vi "纳清电导率_所有参数读取.vi"(8 "error in (no error)":errorcluster caption="错误输入（无错误）", 11 "MB session in":refnum<class "MB_Master.lvclass">) -> (0 "error out":errorcluster caption="错误输出", 2 "输出值":T1 {"波特率" items=["4800", "9600", "19200", "38400", "57600", "115200"]}, 3 "MB session out":refnum<class "MB_Master.lvclass">)   [LabVIEW 2016, in "斯坦道多参数.lvlib"]
uses:
  <vilib>/Plasmionique/MB Master/MB_Master/MB_Master.lvclass
  <vilib>/Plasmionique/MB Master/MB Master.lvlib
  <vilib>/ptbypt/NI_PtbyPt.lvlib
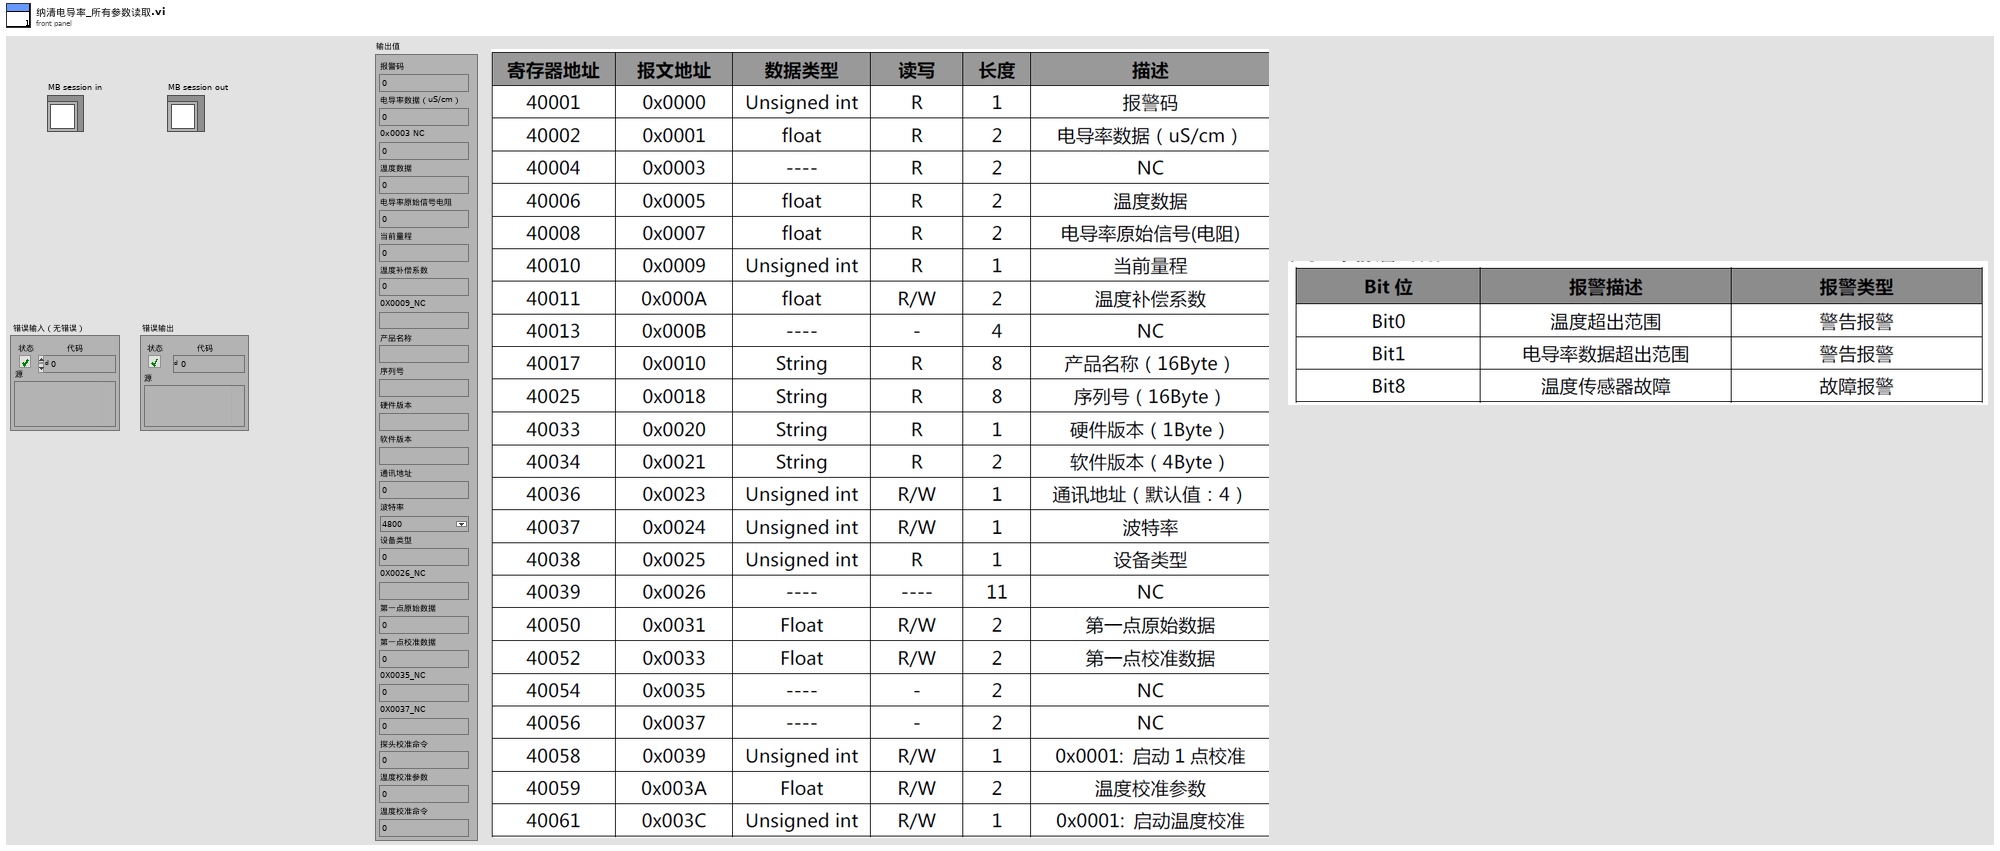
[diagram p1: front panel]
types:
  T1 = cluster{"报警码":u16, "电导率数据（uS/cm）":sgl, "0x0003 NC":sgl, "温度数据":sgl, "电导率原始信号电阻":sgl, "当前量程":u16, "温度补偿系数":sgl, "0X0009_NC":string, "产品名称":string, "序列号":string, "硬件版本":string, "软件版本":string, "通讯地址":u16, "波特率":u16, "设备类型":u16, "0X0026_NC":string, "第一点原始数据":sgl, "第一点校准数据":sgl, "0X0035_NC":sgl, "0X0037_NC":sgl, "探头校准命令":u16, "温度校准参数":sgl, "温度校准命令":u16}
  T2 = cluster{u16, "Filtered x":dbl, "数值":sgl, "数值":sgl, "数值":sgl, u16, "数值":sgl, "类型":string, "类型":string, "类型":string, "类型":string, "类型":string, u16, u16, u16, "类型":string, "数值":sgl, "数值":sgl, "数值":sgl, "数值":sgl, u16, "数值":sgl, u16}
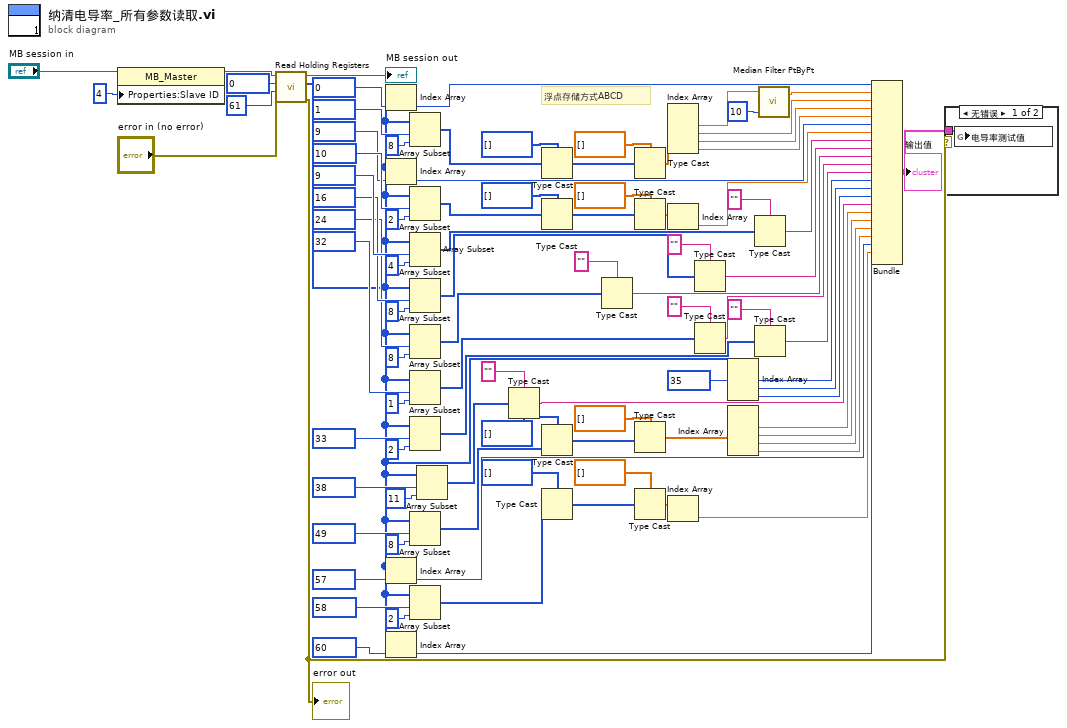
[diagram p0: block diagram]
diagram:
  # "浮点存储方式ABCD"
  n1 = property class="MB_Master"(reference="MB session in", "Properties:Slave ID"=u8 4 ("Slave ID")) -> (reference out=w82:refnum<class "MB_Master.lvclass">)  [unwired: 1 in, 1 out]
  n2 = call <vilib>:"Read Holding Registers.vi"("error in (no error)"="error in (no error)", "quantity"=u16 61, "starting address"=u16 0, "MB session in"=w82) -> ("error out"=w24:errorcluster, "Registers"=w5:u16[], "MB session out"=→"MB session out":refnum<class "MB_Master.lvclass">)  [unwired: 5 in]
  "error out" <- w24
  n3 = Index Array(array=w5, index=u16 0 ("starting address")) -> (element=w90:u16)
  n4 = Index Array(array=w5, index=u16 9 ("starting address")) -> (element=w4:u16)
  n5 = Index Array(array=w5, index=u16 57 ("starting address")) -> (element=w28:u16)
  n6 = Index Array(array=w5, index=u16 60 ("starting address")) -> (element=w25:u16)
  n7 = Array Subset(array=w5, index=u16 1 ("starting address"), length=8 ("长度")) -> (w86:u16[])
  n8 = Array Subset(array=w5, index=u16 10 ("starting address"), length=2 ("长度")) -> (w8:u16[])
  n9 = Array Subset(array=w5, index=u16 9 ("starting address"), length=4 ("长度")) -> (w76:u16[])
  n10 = Array Subset(array=w5, index=u16 16 ("starting address"), length=8 ("长度")) -> (w72:u16[])
  n11 = Array Subset(array=w5, index=u16 24 ("starting address"), length=8 ("长度")) -> (w66:u16[])
  n12 = Array Subset(array=w5, index=u16 32 ("starting address"), length=1 ("长度")) -> (w62:u16[])
  n13 = Array Subset(array=w5, index=u16 33 ("starting address"), length=2 ("长度")) -> (w56:u16[])
  n14 = Array Subset(array=w5, index=u16 49 ("starting address"), length=8 ("长度")) -> (w43:u16[])
  n15 = Array Subset(array=w5, index=u16 58 ("starting address"), length=2 ("长度")) -> (w31:u16[])
  n16 = Array Subset(array=w5, index=u16 38 ("starting address"), length=11 ("长度")) -> (w46:u16[])
  n17 = Type Cast(type="" ("类型"), x=w46) -> (*(type *) &x=w45:string)
  n18 = Type Cast(type=u32[] [] ("数组 2"), x=w86) -> (*(type *) &x=w23:u32[])
  n19 = Type Cast(type=u32[] [] ("数组 2"), x=w8) -> (*(type *) &x=w12:u32[])
  n20 = Type Cast(type=u32[] [] ("数组 2"), x=w43) -> (*(type *) &x=w41:u32[])
  n21 = Type Cast(type=u32[] [] ("数组 2"), x=w31) -> (*(type *) &x=w33:u32[])
  n22 = Type Cast(type="" ("类型"), x=w66) -> (*(type *) &x=w64:string)
  n23 = Type Cast(type=sgl[] [] ("数组 2"), x=w23) -> (*(type *) &x=w85:sgl[])
  n24 = Type Cast(type=sgl[] [] ("数组 2"), x=w12) -> (*(type *) &x=w11:sgl[])
  n25 = Type Cast(type=sgl[] [] ("数组 2"), x=w41) -> (*(type *) &x=w38:sgl[])
  n26 = Type Cast(type=sgl[] [] ("数组 2"), x=w33) -> (*(type *) &x=w36:sgl[])
  n27 = Index Array(array=w85) -> (element #1=w2:sgl, element #2=w80:sgl, element #3=w20:sgl, element #4=w19:sgl)  [unwired: 4 in]
  n28 = Index Array(array=w11) -> (element=w7:sgl)  [unwired: 1 in]
  n29 = Index Array(array=w36) -> (element=w27:sgl)  [unwired: 1 in]
  n30 = Type Cast(type="" ("类型"), x=w72) -> (*(type *) &x=w69:string)
  n31 = Type Cast(type="" ("类型"), x=w62) -> (*(type *) &x=w59:string)
  n32 = Index Array(array=w5, index #1=u16 35 ("starting address")) -> (element #1=w52:u16, element #2=w51:u16, element #3=w50:u16)  [unwired: 2 in]
  n33 = Index Array(array=w38) -> (element #1=w37:sgl, element #2=w18:sgl, element #3=w17:sgl, element #4=w16:sgl)  [unwired: 4 in]
  n34 = Type Cast(type="" ("类型"), x=w76) -> (*(type *) &x=w74:string)
  n35 = Type Cast(type="" ("类型"), x=w56) -> (*(type *) &x=w54:string)
  n36 = call <vilib>:"Median Filter PtByPt.vi"("rank"=10, "x"=w2) -> ("Filtered x"=w1:dbl)  [unwired: 2 in, 1 out]
  n37 = Bundle(w90, "Filtered x"=w1, "数值"=w80, "数值"=w20, "数值"=w19, w4, "数值"=w7, "类型"=w74, "类型"=w69, "类型"=w64, "类型"=w59, "类型"=w54, w52, w51, w50, "类型"=w45, "数值"=w37, "数值"=w18, "数值"=w17, "数值"=w16, w28, "数值"=w27, w25) -> (w15:T2)  [unwired: 1 in]
  "输出值" <- w15
  n38 = case shown="无错误" w24 {
    tunnel: w15 -> [w93 _]
    frame No Error {
      n39 = global write "纳清过程全局变量.vi" "电导率测试值"(w93) -> ()
    }
    frame Error {
    }
  }
